vi "Disconnect.vi"(8 "error in (no error)":errorcluster, 11 "B&K Precision 9120 series in":refnum<class "B&K Precision 9120 series.lvclass">) -> (0 "error out":errorcluster, 3 "B&K Precision 9120 series out":refnum<class "B&K Precision 9120 series.lvclass">)   [LabVIEW 2014, in "B&K Precision 9120 series.lvclass"]
uses:
  B&K Precision 9120 series.lvclass
  B&K Precision 9120 series.lvclass/B&K Precision 9120 series.ctl
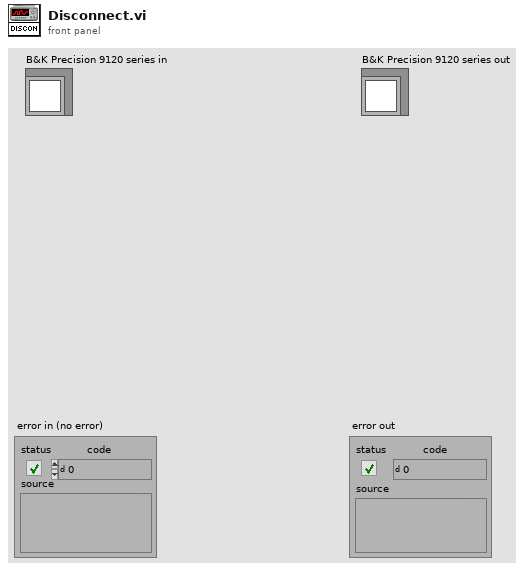
[diagram p1: front panel]
types:
  T1 = typedef "B&K Precision 9120 series.lvclass/Serial_Config.ctl" = cluster{"Baud":u32, "Flow Ctl":u16, "COM port":refnum<visa-resource-name>, "Parity":u16}
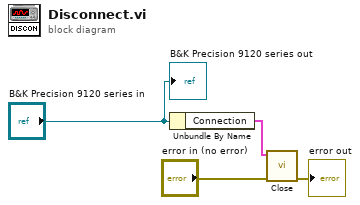
[diagram p0: block diagram]
diagram:
  n1 = Unbundle By Name("B&K Precision 9120 series in") -> ("Connection"=w2:T1)
  n2 = call "Close.vi"("error in (no error)"="error in (no error)", "Connection"=w2) -> ("error out"=→"error out":errorcluster)  [unwired: 9 in]
  "B&K Precision 9120 series out" <- "B&K Precision 9120 series in"
